vi "Get Device Serial Number.vi"(0 "Session Handle in":T1, 11 "error in (no error)":errorcluster) -> (4 "Session Handle out":T1, 6 "Failure Reason":string, 8 "Failure?":bool, 10 "Serial Number":string, 15 "error out":errorcluster)   [LabVIEW 2015, in "Oil.lvclass"]
uses:
  Oil.lvclass
  Typedefs/Session Handle.ctl
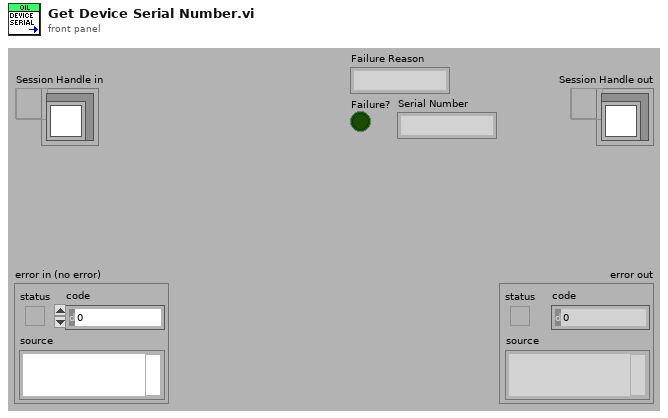
[diagram p1: front panel]
types:
  T1 = typedef "Oil.lvclass/Session Handle.ctl" = refnum<data-value>
  T2 = typedef "XNET Frame CAN.ctl" = cluster{"timestamp":timestamp, "payload":u8[], "identifier":u32, "type":T3, "extended?":bool, "echo?":bool}
  T3 = typedef "XNET Frame Type CAN.ctl" = u8
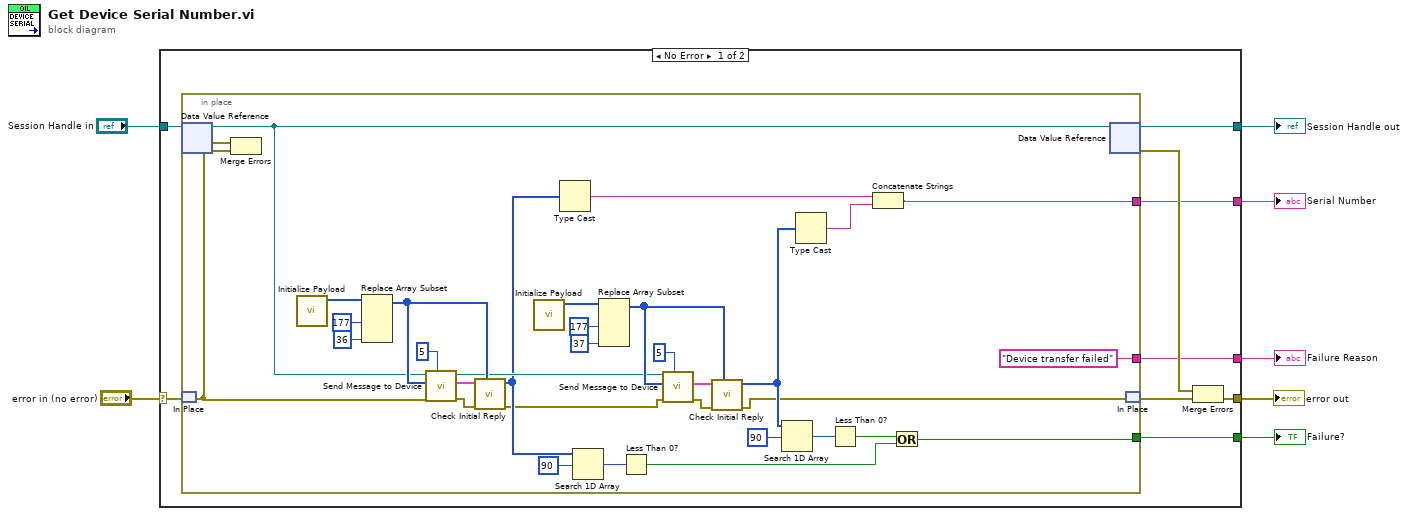
[diagram p0: block diagram]
diagram:
  n1 = case shown="No Error" "error in (no error)" {
    selector: "error in (no error)" -> [w11 w50]
    tunnel: "Session Handle in" -> [w16 w51]
    tunnel: [w15 w51] -> w6
    tunnel: [w12 w50] -> w5
    tunnel: [w10 _] -> w3
    tunnel: [w9 _] -> w2
    tunnel: [w8 _] -> w1
    frame No Error {
      n2 = in-place {
        in-place-border: ["Device transfer failed"] -> w10
        in-place-border: [w27] -> w9
        in-place-border: [w25] -> w8
        n3 = in-place-dvr #1(w16) -> (w41:refnum<class "Oil.lvclass">, w49:errorcluster)
        n4 = in-place-match #2(w11) -> (w42:errorcluster)
        n5 = Merge Errors(w42, w49) -> ()  [unwired: 1 out]
        n6 = call "Initialize Payload.vi"() -> ("Initial Payload"=w48:u8[])  [unwired: 11 in]
        n7 = Replace Array Subset(array=w48, new element #1=u8 177 ("new element/subarray"), new element #2=u8 36 ("new element/subarray")) -> (w43:u8[])  [unwired: 2 in]
        n8 = call "Send Message to Device.vi"("Number of Retries"=5, "error in (no error)"=w42, "payload"=w43, "CAN Comm In"=w41) -> ("error out"=w20:errorcluster, "Reply"=w44:T2[], "CAN Comm Out"=w34:refnum<class "Oil.lvclass">)  [unwired: 5 in]
        n9 = call "Check Initial Reply.vi"("Write Message"=w43, "error in (no error)"=w20, "Reply"=w44) -> ("error out"=w19:errorcluster, "Data Packet 2"=w24:u8[])  [unwired: 5 in, 2 out]
        n10 = call "Initialize Payload.vi"() -> ("Initial Payload"=w35:u8[])  [unwired: 11 in]
        n11 = Type Cast(x=w24) -> (*(type *) &x=w23:string)  [unwired: 1 in]
        n12 = Search 1D Array(1D array=w24, element=u8 90 ("new element/subarray")) -> (index of element=w32:i32)  [unwired: 1 in]
        n13 = Replace Array Subset(array=w35, new element #1=u8 177 ("new element/subarray"), new element #2=u8 37 ("new element/subarray")) -> (w40:u8[])  [unwired: 2 in]
        n14 = Less Than 0?(x=w32) -> (x < 0?=w28:bool)
        n15 = call "Send Message to Device.vi"("Number of Retries"=5, "error in (no error)"=w19, "payload"=w40, "CAN Comm In"=w34) -> ("error out"=w18:errorcluster, "Reply"=w39:T2[])  [unwired: 5 in, 1 out]
        n16 = call "Check Initial Reply.vi"("Write Message"=w40, "error in (no error)"=w18, "Reply"=w39) -> ("error out"=w17:errorcluster, "Data Packet 2"=w22:u8[])  [unwired: 5 in, 2 out]
        n17 = Search 1D Array(1D array=w22, element=u8 90 ("new element/subarray")) -> (index of element=w31:i32)  [unwired: 1 in]
        n18 = Type Cast(x=w22) -> (*(type *) &x=w21:string)  [unwired: 1 in]
        n19 = Less Than 0?(x=w31) -> (x < 0?=w29:bool)
        n20 = Concatenate Strings(w23, w21) -> (w25:string)
        n21 = Or(x=w29, y=w28) -> (x .or. y?=w27:bool)
        n22 = in-place-dvr #1(w41) -> (w15:T1, w13:errorcluster)
        n23 = in-place-match #2(w17) -> (w14:errorcluster)
      }
      n24 = Merge Errors(w13, w14) -> (w12:errorcluster)
    }
    frame Error {
    }
  }
  "Session Handle out" <- w6
  "error out" <- w5
  "Failure Reason" <- w3
  "Failure?" <- w2
  "Serial Number" <- w1
